vi "Initialize_mod.vi"(8 "error in (no error)":errorcluster, 9 "Reset (True)":bool=TRUE, 10 "ID Query (True)":bool=TRUE, 11 "VISA resource name":refnum<visa-resource-name>) -> (0 "error out":errorcluster, 3 "VISA resource name out":refnum<visa-resource-name>)   [LabVIEW 2015]
doc: "Establishes communication with an oscilloscope. This VI optionally performs an instrument identification query and/or resets the oscilloscope. The Initialize VI also configures the oscilloscope to a default state that other instrument driver operations require.\nRun this VI before running other instrument driver VIs for the oscilloscope. You generally need to call the Initialize VI only once, at the beginning of an application."
uses:
  Extended User Data_mod.ctl
  Tektronix DPO MSO 2000 4000 Series/Tektronix DPO MSO 2000 4000 Series.lvlib
panel:
  # "(C) 2006 - 2014. National Instruments Corporation. ALL RIGHTS RESERVED."
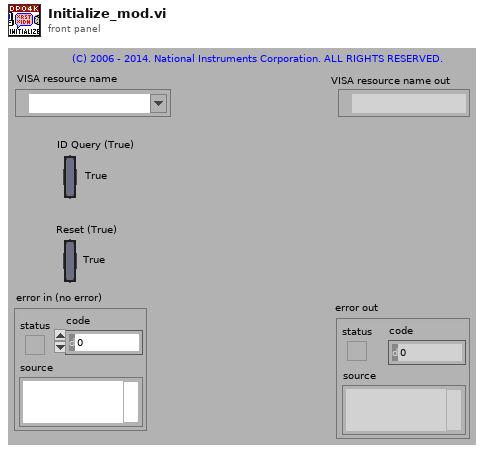
[diagram p1: front panel]
types:
  T1 = typedef "Extended User Data_mod.ctl" = cluster{"DPO MSO Series Model":u16}
  T2 = enum16{"DPO4104", "DPO4054", "DPO4034", "DPO4032"}
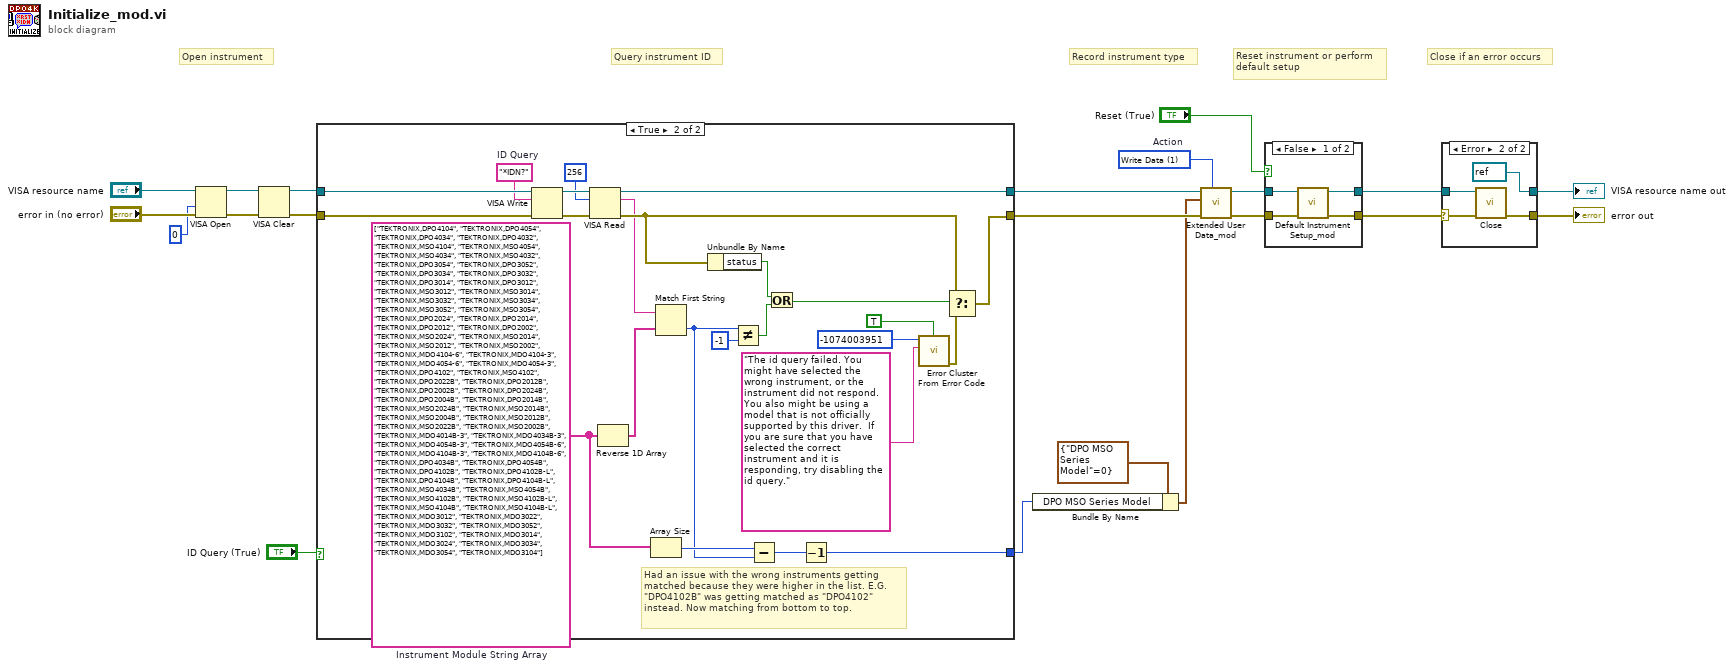
[diagram p0: block diagram]
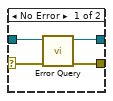
[diagram p2: hidden frame]
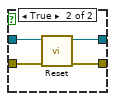
[diagram p3: hidden frame]
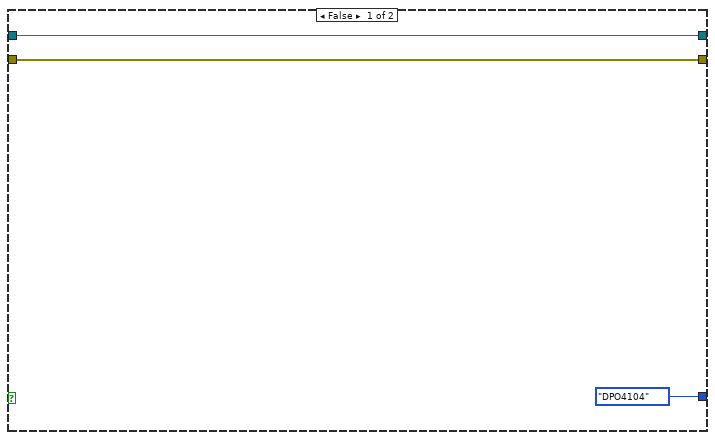
[diagram p4: hidden frame]
diagram:
  w6 = 1 items=["Read Data", "Write Data", "Clear Data", "Clear ALL Data"]  # Action
  # "Record instrument type"
  # "Close if an error occurs"
  # "Query instrument ID"
  # "Reset instrument or perform\ndefault setup"
  # "Open instrument"
  n1 = VISA Open(access mode=u32 0, error in (no error)="error in (no error)", VISA resource name="VISA resource name") -> (VISA resource name=w9:refnum<visa-resource-name>, error out=w17:errorcluster)  [unwired: 2 in]
  n2 = VISA Clear(VISA resource name=w9, error in (no error)=w17) -> (VISA resource name out=w12:refnum<visa-resource-name>, error out=w11:errorcluster)
  n3 = case shown="True" "ID Query (True)" {
    tunnel: [w23 w48] -> w7
    tunnel: [w24 w45] -> w8
    tunnel: w12 -> [w24 w46]
    tunnel: w11 -> [w23 w47]
    tunnel: [T2."DPO4104" ("Instrument Module") w25] -> w4
    frame False {
    }
    frame True {
      w29 = string[] ["TEKTRONIX,DPO4104", "TEKTRONIX,DPO4054", "TEKTRONIX,DPO4034", "TEKTRONIX,DPO4032", "TEKTRONIX,MSO4104", "TEKTRONIX,MSO4054", "TEKTRONIX,MSO4034", "TEKTRONIX,MSO4032", "TEKTRONIX,DPO3054", "TEKTRONIX,DPO3052", "TEKTRONIX,DPO3034", "TEKTRONIX,DPO3032", "TEKTRONIX,DPO3014", "TEKTRONIX,DPO3012", "TEKTRONIX,MSO3012", "TEKTRONIX,MSO3014", "TEKTRONIX,MSO3032", "TEKTRONIX,MSO3034", "TEKTRONIX,MSO3052", "TEKTRONIX,MSO3054", "TEKTRONIX,DPO2024", "TEKTRONIX,DPO2014", "TEKTRONIX,DPO2012", "TEKTRONIX,DPO2002", "TEKTRONIX,MSO2024", "TEKTRONIX,MSO2014", "TEKTRONIX,MSO2012", "TEKTRONIX,MSO2002", "TEKTRONIX,MDO4104-6", "TEKTRONIX,MDO4104-3", "TEKTRONIX,MDO4054-6", "TEKTRONIX,MDO4054-3", "TEKTRONIX,DPO4102", "TEKTRONIX,MSO4102", "TEKTRONIX,DPO2022B", "TEKTRONIX,DPO2012B", "TEKTRONIX,DPO2002B", "TEKTRONIX,DPO2024B", "TEKTRONIX,DPO2004B", "TEKTRONIX,DPO2014B", "TEKTRONIX,MSO2024B", "TEKTRONIX,MSO2014B", "TEKTRONIX,MSO2004B", "TEKTRONIX,MSO2012B", "TEKTRONIX,MSO2022B", "TEKTRONIX,MSO2002B", "TEKTRONIX,MDO4014B-3", "TEKTRONIX,MDO4034B-3", "TEKTRONIX,MDO4054B-3", "TEKTRONIX,MDO4054B-6", "TEKTRONIX,MDO4104B-3", "TEKTRONIX,MDO4104B-6", "TEKTRONIX,DPO4034B", "TEKTRONIX,DPO4054B", "TEKTRONIX,DPO4102B", "TEKTRONIX,DPO4102B-L", "TEKTRONIX,DPO4104B", "TEKTRONIX,DPO4104B-L", "TEKTRONIX,MSO4034B", "TEKTRONIX,MSO4054B", "TEKTRONIX,MSO4102B", "TEKTRONIX,MSO4102B-L", "TEKTRONIX,MSO4104B", "TEKTRONIX,MSO4104B-L", "TEKTRONIX,MDO3012", "TEKTRONIX,MDO3022", "TEKTRONIX,MDO3032", "TEKTRONIX,MDO3052", "TEKTRONIX,MDO3102", "TEKTRONIX,MDO3014", "TEKTRONIX,MDO3024", "TEKTRONIX,MDO3034", "TEKTRONIX,MDO3054", "TEKTRONIX,MDO3104"]  # Instrument Module String Array
      w41 = "*IDN?"  # ID Query
      # "Had an issue with the wrong instruments getting\nmatched because they were higher in the list. E.G.\n\"DPO4102B\" was getting matched as \"DPO4102\"\ninstead. Now matching from bottom to top."
      n4 = VISA Write(VISA resource name=w46, write buffer=w41, error in (no error)=w47) -> (VISA resource name out=w44:refnum<visa-resource-name>, error out=w43:errorcluster)  [unwired: 1 out]
      n5 = VISA Read(VISA resource name=w44, byte count=u32 256, error in (no error)=w43) -> (VISA resource name out=w45:refnum<visa-resource-name>, read buffer=w35:string, error out=w36:errorcluster)  [unwired: 1 out]
      n6 = Reverse 1D Array(array=w29) -> (reversed array=w30:string[])
      n7 = Array Size(array=w29) -> (size(s)=w28:i32)
      n8 = Match First String(2:w30, 3:w35) -> (0:w27:i32)  [unwired: 1 out]
      n9 = Unbundle By Name(w36) -> ("status"=w33:bool)
      n10 = Not Equal?(x=w27, y=-1) -> (x != y?=w32:bool)
      n11 = Subtract(x=w28, y=w27) -> (x-y=w26:i32)
      n12 = Or(x=w33, y=w32) -> (x .or. y?=w31:bool)
      n13 = Decrement(x=w26) -> (x-1=w25:i32)
      n14 = call <vilib>:"Error Cluster From Error Code.vi"("show call chain? (False)"=TRUE, "error message (\"\")"="The id query failed. You might have selected the wrong instrument, or the instrument did not respond.  You also might be using a model that is not officially supported by this driver.  If you are sure that you have selected the correct instrument and it is responding, try disabling the id query." ("Source (VI Name)"), "error code (0)"=-1074003951 ("Code")) -> ("error out"=w40:errorcluster)  [unwired: 6 in]
      n15 = Select(t=w36, s=w31, f=w40) -> (s? t:f=w48:errorcluster)
    }
  }
  n16 = Bundle By Name(cluster=T1 {"DPO MSO Series Model"=0} ("User Data In"), "DPO MSO Series Model"=w4) -> (w3:T1)
  n17 = call "Extended User Data_mod.vi"("Action (1: Write Data)"=w6, "error in (no error)"=w7, "User Data In"=w3, "VISA resource name"=w8) -> ("error out"=w1:errorcluster, "VISA resource name out"=w2:refnum<visa-resource-name>)  [unwired: 5 in, 1 out]
  n18 = case shown="False" "Reset (True)" {
    tunnel: w1 -> [w51 w53]
    tunnel: [w50 w56] -> w13
    tunnel: w2 -> [w52 w54]
    tunnel: [w49 w55] -> w14
    frame False {
      n19 = call "Default Instrument Setup_mod.vi"("error in (no error)"=w51, "VISA resource name"=w52) -> ("error out"=w50:errorcluster, "VISA resource name out"=w49:refnum<visa-resource-name>)  [unwired: 8 in]
    }
    frame True {
      n20 = call "Reset.vi"("error in (no error)"=w53, "VISA resource name"=w54) -> ("error out"=w56:errorcluster, "VISA resource name out"=w55:refnum<visa-resource-name>)  [unwired: 8 in]
    }
  }
  n21 = case shown="Error" w13 {
    selector: w13 -> [w58 w62]
    tunnel: w14 -> [w57 w63]
    tunnel: [w60 refnum<visa-resource-name> refnum ("VISA resource name out")] -> w16
    tunnel: [w59 w64] -> w15
    frame No Error {
      n22 = call "Error Query.vi"("error in (no error)"=w58, "VISA resource name"=w57) -> ("error out"=w59:errorcluster, "VISA resource name out"=w60:refnum<visa-resource-name>)  [unwired: 6 in, 2 out]
    }
    frame Error {
      n23 = call "Close.vi"("error in (no error)"=w62, "VISA resource name"=w63) -> ("error out"=w64:errorcluster)  [unwired: 9 in]
    }
  }
  "VISA resource name out" <- w16
  "error out" <- w15
